vi "HAM Digital Radio.vi"() -> ()   [LabVIEW 2013]
uses:
  STYPS/HDR - Queues.ctl
panel:
  in  "Queues":T1
  in  "Global_Event":cluster{"CMD":string}
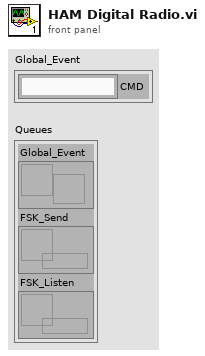
[diagram p1: front panel]
types:
  T1 = typedef "HDR - Queues.ctl" = cluster{"Global_Event":refnum<user-event>, "FSK_Send":refnum<queue>, "FSK_Listen":refnum<queue>}
  T2 = enum32{"Invalid", "Standard", "Closed", "Hidden", "Minimized", "Maximized"}
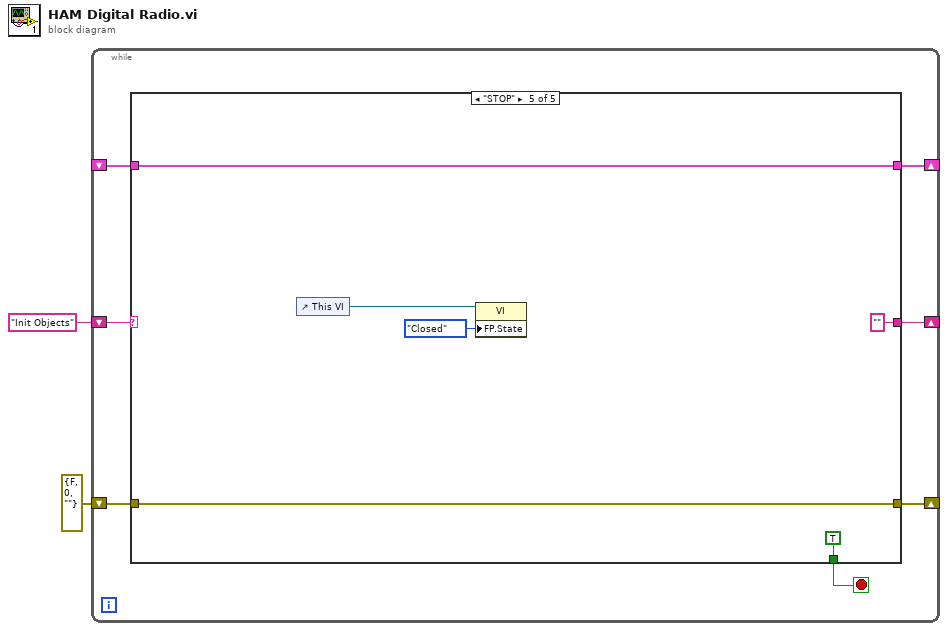
[diagram p0: block diagram]
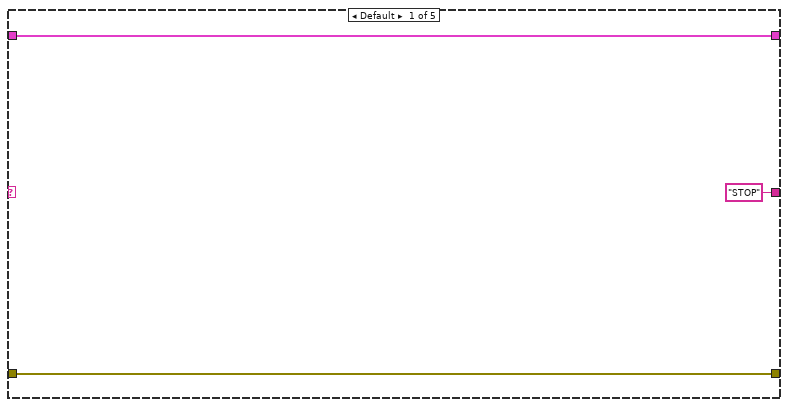
[diagram p2: hidden frame]
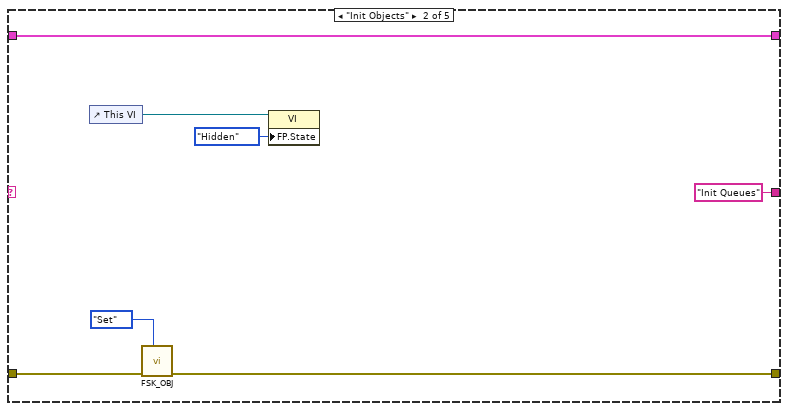
[diagram p3: hidden frame]
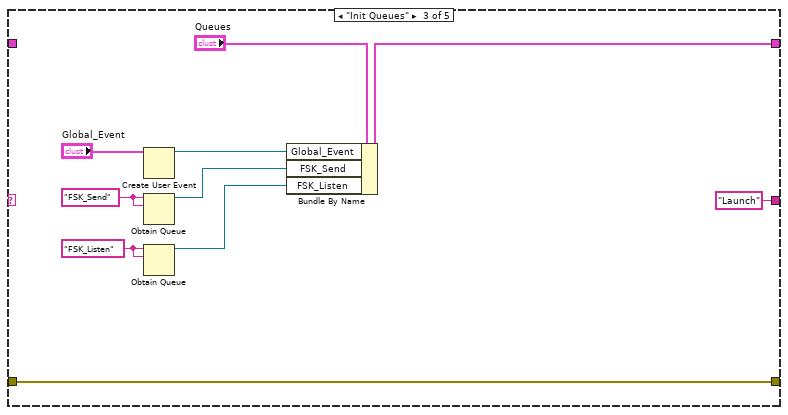
[diagram p4: hidden frame]
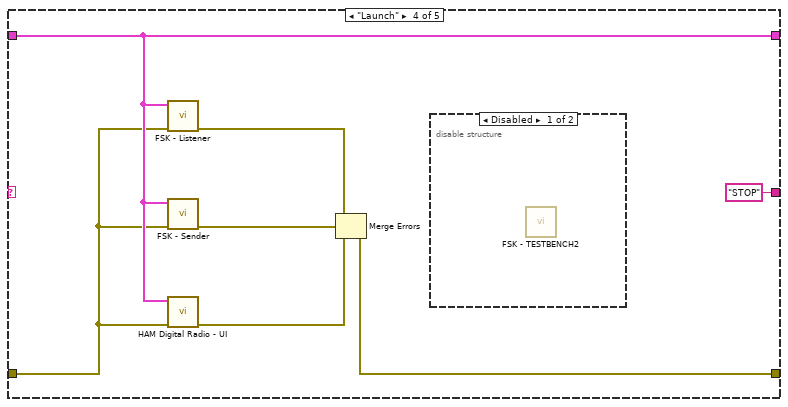
[diagram p5: hidden frame]
diagram:
  n1 = while {
    shift-right: [w8] -> _
    shift-left: errorcluster {"status"=FALSE, "code"=0, "source"=""} ("error out") -> [w7]
    shift-right: [w4] -> _
    shift-left: _ -> [w3]
    shift-right: [w6] -> _
    shift-left: "Init Objects" -> [w9]
    stop <- w5 stop-if-true
    n2 = case shown="\"STOP\"" w9 {
      tunnel: [w12 w19 w28 w33 w41] -> w8
      tunnel: w7 -> [w12 w18 w28 w31 w41]
      tunnel: ["STOP" "Init Queues" "Launch" "STOP" ""] -> w6
      tunnel: [_ _ _ _ TRUE] -> w5
      tunnel: [w10 w15 w24 w32 w39] -> w4
      tunnel: w3 -> [w10 w15 _ w32 w39]
      frame Default {
      }
      frame "Init Objects" {
        n3 = control-ref of="This VI"() -> (w14:refnum<vi>)
        n4 = call "FSK_OBJ.vi"("Mode"=enum16{"Get", "Set"}."Set", "error in"=w18) -> ("error out"=w19:errorcluster)  [unwired: 8 in, 1 out]
        n5 = property class="VI"(reference=w14, "FP.State"=T2."Hidden" ("Front Panel Window:State")) -> ()  [unwired: 1 in, 2 out]
      }
      frame "Init Queues" {
        w22 = "FSK_Listen" ("name (unnamed)")
        w27 = "FSK_Send" ("name (unnamed)")
        n6 = Create User Event(user event datatype="Global_Event") -> (user event=w23:refnum<user-event>)  [unwired: 1 in, 1 out]
        n7 = Obtain Queue(name (unnamed)=w27, element data type=w27) -> (queue out=w21:refnum<queue>)  [unwired: 3 in, 2 out]
        n8 = Obtain Queue(name (unnamed)=w22, element data type=w22) -> (queue out=w20:refnum<queue>)  [unwired: 3 in, 2 out]
        n9 = Bundle By Name(cluster="Queues", "Global_Event"=w23, "FSK_Send"=w21, "FSK_Listen"=w20) -> (w24:T1)
      }
      frame "Launch" {
        n10 = call "FSK - Listener.vi"("error in (no error)"=w31, "Queues"=w32) -> ("error out"=w34:errorcluster)  [unwired: 9 in]
        n11 = call "FSK - Sender.vi"("error in (no error)"=w31, "Queues"=w32) -> ("error out"=w35:errorcluster)  [unwired: 9 in]
        n12 = call "HAM Digital Radio - UI.vi"("error in (no error)"=w31, "Queues"=w32) -> ("error out"=w30:errorcluster)  [unwired: 9 in]
        n13 = Merge Errors(w34, w35, w30) -> (w33:errorcluster)
        n14 = disable-structure shown="Disabled" {
          frame Disabled {
            n15 = call "FSK - TESTBENCH2.vi"() -> ()  [unwired: 12 in]
          }
          frame Enabled {
          }
        }
      }
      frame "STOP" {
        n16 = control-ref of="This VI"() -> (w38:refnum<vi>)
        n17 = property class="VI"(reference=w38, "FP.State"=T2."Closed" ("Front Panel Window:State")) -> ()  [unwired: 1 in, 2 out]
      }
    }
  }
